vi "3D Shape Test Bench.vi"() -> ()   [LabVIEW 2017]
uses:
  Controls/Room Dimensions.ctl
  Controls/Probe Dimensions.ctl
  Controls/Frame Grabber Data.ctl
  <vilib>/userdefined/High Color/IMAQdx.ctl
  <vilib>/vision/Image Controls.llb/IMAQ Image.ctl
  <vilib>/vision/Avi.llb/IMAQ AVI2 Refnum.ctl
  Controls/Rigid Body Info.ctl
  Controls/Position.ctl
  Controls/Orientation.ctl
  <vilib>/robotics/Kinematics/RotateX.vi
  <vilib>/robotics/Kinematics/RotateY.vi
  <vilib>/robotics/Kinematics/RotateZ.vi
  <vilib>/Analysis/baseanly.llb/A x B.vi
  <vilib>/Analysis/baseanly.llb/Real A x B.vi
  <vilib>/picture/3D Picture Control/NI_3D Picture Control.lvlib
  <vilib>/robotics/Kinematics/NI_Kinematics.lvlib
panel:
  in  "Frame Grabber Data In":T1={"Camera Session"="", "Frame"="frame", "AVI Refnum"=refnum, "Codecs"=["Cinepak Codec by Radius", "Intel IYUV codec", "Microsoft Video 1", "FF Video Codec 1 (FFV1) (NI Vision)", "Motion JPEG (NI Vision)", "Y800 Uncompressed Grey Scale (NI Vision)", "YUV 4:2:0 Planar (NI Vision)"], "Frame number"=0, "OptiTrack Refnum"=refnum, "Tick Count"=0, "Probe Object"=refnum, "Playback Probe Data"=[], "Rigid Body"={"Position"={"x (mm)"=0.0, "y (mm)"=0.0, "z (mm)"=0.0}, "Orientation"={"Pitch (rad)"=0.0, "Yaw (rad)"=0.0, "Roll (rad)"=0.0}, "Tracked?"=FALSE}, "Number of frames to playback"=0, "Playback FPS"=0, "Camera connected?"=FALSE, "Scene"=refnum, "Frame Number Refnum"=refnum}
  in  "Probe Dimensions":T8={"Probe Width"=1.0, "Probe Depth"=1.2, "Probe Height"=2.0}
  in  "Room Dimensions":T9={"Room Width"=100.0, "Room Depth"=100.0, "Room Height"=100.0}
  out "Error Out":errorcluster={"status"=TRUE, "code"=1088, "source"="Property Node (arg 2) in NI_3D Picture Control.lvlib:Create Box.vi->Create 3D Shapes.vi->3D Shape Test Bench.vi"}
  in  "Error In":errorcluster
  in  "Initial Probe Position":cluster{"X":sgl, "Y":sgl, "Z":sgl}
  in  "Orientation":cluster{"X":sgl, "Y":sgl, "Z":sgl}
  in  "Stop Button":bool
  out "Scene":refnum<vi>(3d-picture)
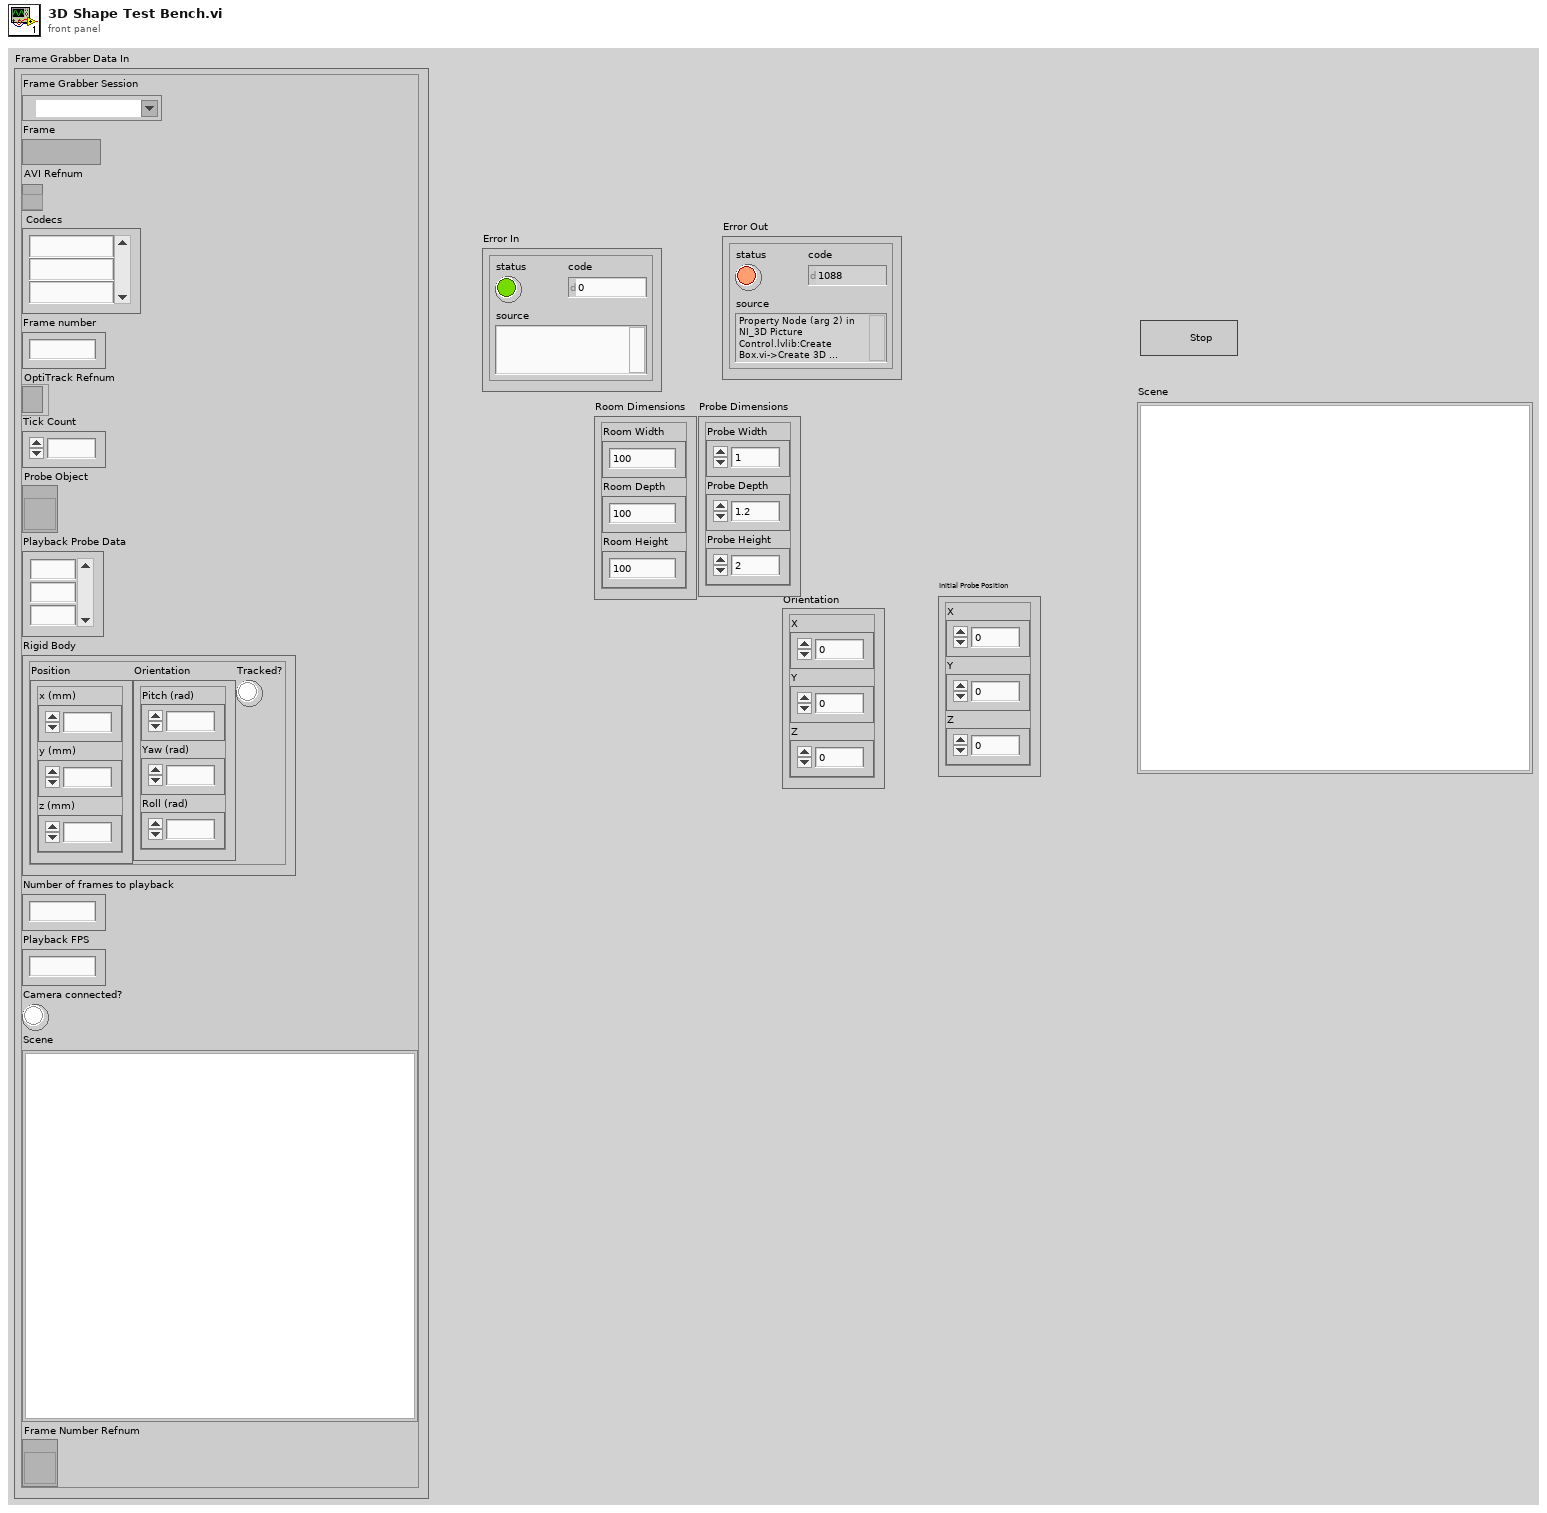
[diagram p1: front panel]
types:
  T1 = typedef "Frame Grabber Data.ctl" = cluster{"Camera Session":T2, "Frame":T3, "AVI Refnum":T4, "Codecs":string[], "Frame number":u32, "OptiTrack Refnum":refnum<file>, "Tick Count":u32, "Probe Object":refnum<vi>, "Playback Probe Data":dbl[][], "Rigid Body":T5, "Number of frames to playback":u32, "Playback FPS":u32, "Camera connected?":bool, "Scene":refnum<vi>, "Frame Number Refnum":refnum<vi>}
  T2 = typedef "IMAQdx.ctl" = refnum<k21>
  T3 = typedef "IMAQ Image.ctl" = refnum<image>
  T4 = typedef "IMAQ AVI2 Refnum.ctl" = refnum<k20>
  T5 = typedef "Rigid Body Info.ctl" = cluster{"Position":T6, "Orientation":T7, "Tracked?":bool}
  T6 = typedef "Position.ctl" = cluster{"x (mm)":sgl, "y (mm)":sgl, "z (mm)":sgl}
  T7 = typedef "Orientation.ctl" = cluster{"Pitch (rad)":sgl, "Yaw (rad)":sgl, "Roll (rad)":sgl}
  T8 = typedef "Probe Dimensions.ctl" = cluster{"Probe Width":sgl, "Probe Depth":sgl, "Probe Height":sgl}
  T9 = typedef "Room Dimensions.ctl" = cluster{"Room Width":dbl, "Room Depth":dbl, "Room Height":dbl}
  T10 = typedef "NI_Matrix.lvlib/RealMatrix.ctl" = dbl[][]
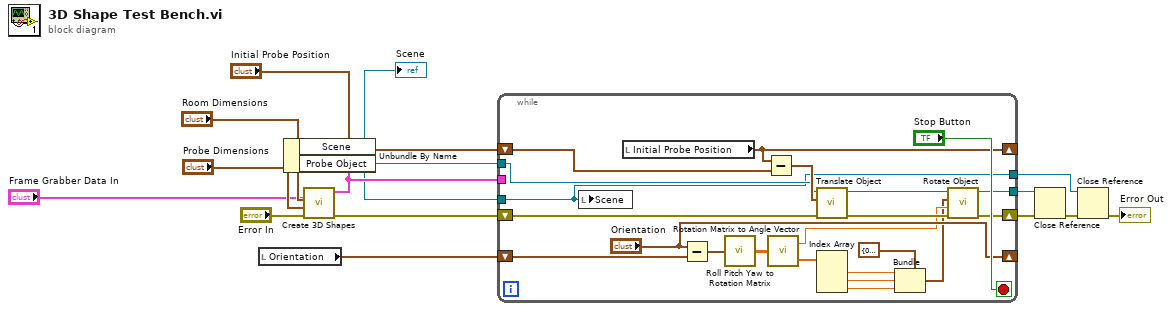
[diagram p0: block diagram]
diagram:
  n1 = local read "Orientation"() -> (w15:cluster{"X":sgl, "Y":sgl, "Z":sgl})
  n2 = call "Create 3D Shapes.vi"("error in (no error)"="Error In", "Probe Dimensions"="Probe Dimensions", "Room Dimensions"="Room Dimensions", "Frame Grabber Data In"="Frame Grabber Data In") -> ("error out"=w14:errorcluster, "Frame Grabber Data Out"=w4:T1)  [unwired: 6 in]
  n3 = Unbundle By Name(w4) -> ("Scene"=w3:refnum<vi>, "Probe Object"=w2:refnum<vi>)
  "Scene" <- w3
  n4 = while {
    shift-right: ["Orientation"] -> _
    shift-left: w15 -> [w33]
    shift-right: [w18] -> _
    shift-left: "Initial Probe Position" -> [w30]
    shift-right: [w34] -> w12
    shift-left: w14 -> [w36]
    tunnel: w4 -> [_]
    tunnel: [w31] -> w13
    tunnel: w3 -> [w16]
    tunnel: w2 -> [w17]
    tunnel: [w16] -> w1
    stop <- "Stop Button" stop-if-true
    n5 = local write "Scene"(w16) -> ()
    n6 = local read "Initial Probe Position"() -> (w18:cluster{"X":sgl, "Y":sgl, "Z":sgl})
    n7 = Subtract(x="Orientation", y=w33) -> (x-y=w25:cluster{"X":sgl, "Y":sgl, "Z":sgl})
    n8 = call <vilib>:"Roll Pitch Yaw to Rotation Matrix.vi"("angles"=w25) -> ("rotation matrix"=w27:T10)
    n9 = Subtract(x=w18, y=w30) -> (x-y=w29:cluster{"X":sgl, "Y":sgl, "Z":sgl})
    n10 = call <vilib>:"Rotation Matrix to Angle Vector.vi"("rotation matrix"=w27) -> ("angle"=w26:dbl, "vector"=w23:dbl[])
    n11 = call <vilib>:"Translate Object.vi"("error in (no error)"=w36, "Translation"=w29, "Scene.Object In"=w17) -> ("error out"=w35:errorcluster, "Scene.Object Out"=w32:refnum<vi>)  [unwired: 7 in]
    n12 = Index Array(array=w23) -> (element #1=w20:dbl, element #2=w21:dbl, element #3=w22:dbl)  [unwired: 3 in]
    n13 = Bundle(cluster=cluster{"X":sgl, "Y":sgl, "Z":sgl} {"X"=0.0, "Y"=0.0, "Z"=0.0} ("Axis"), "X"=w20, "Y"=w21, "Z"=w22) -> (w19:cluster{"X":sgl, "Y":sgl, "Z":sgl})
    n14 = call <vilib>:"Rotate Object.vi"("error in (no error)"=w35, "Angle"=w26, "Axis"=w19, "Scene.Object In"=w32) -> ("error out"=w34:errorcluster, "Scene.Object Out"=w31:refnum<vi>)  [unwired: 6 in]
  }
  n15 = Close Reference(reference=w13, error in (no error)=w12) -> (error out=w11:errorcluster)
  n16 = Close Reference(reference=w1, error in (no error)=w11) -> (error out=→"Error Out":errorcluster)
